vi "周期拟合倒时反应性.vi"() -> ()   [LabVIEW 2020]
uses:
  <vilib>/Utility/miscctls.llb/LVAnnotationListTypeDef.ctl
  <vilib>/Analysis/NI_AALPro.lvlib
panel:
  out "反应性相对偏差":dbl[](array[numeric]) caption="相对偏差 (%)"
  out "最小二乘周期":dbl[](array[numeric]) caption="最小二乘法拟合 (s)"
  out "广义指数周期":dbl[](array[numeric]) caption="广义指数拟合 (s)"
  out "实测平均反应性":dbl[](array[numeric]) caption="实测平均值 (pcm)"
  out "周期法反应性":dbl[](array[numeric]) caption="周期法 (pcm)"
  out "采样间隔":dbl
  out "开始时间":timestamp
  in  "打开文件":bool
  out "历史波形图":cluster{dbl, dbl, dbl[][]}(graph)
  out "左选标时刻":timestamp caption="左选标时刻：" format="%<%.2X %x>T"
  out "数据点数":i32 caption="选中的数据点数："
  out "反应性记录表":string[][](table) caption="计算结果记录表"
  in  "保存表格":bool
  in  "添加记录":bool
  out "提示信息":string="打开文件后，拖动波形图中的游标选取临界段、动态段和终端段数据进行计算。"
  out "文件信息":string
  # "周期计算结果"
  # "反应性计算结果"
  # "坐标轴与图例"
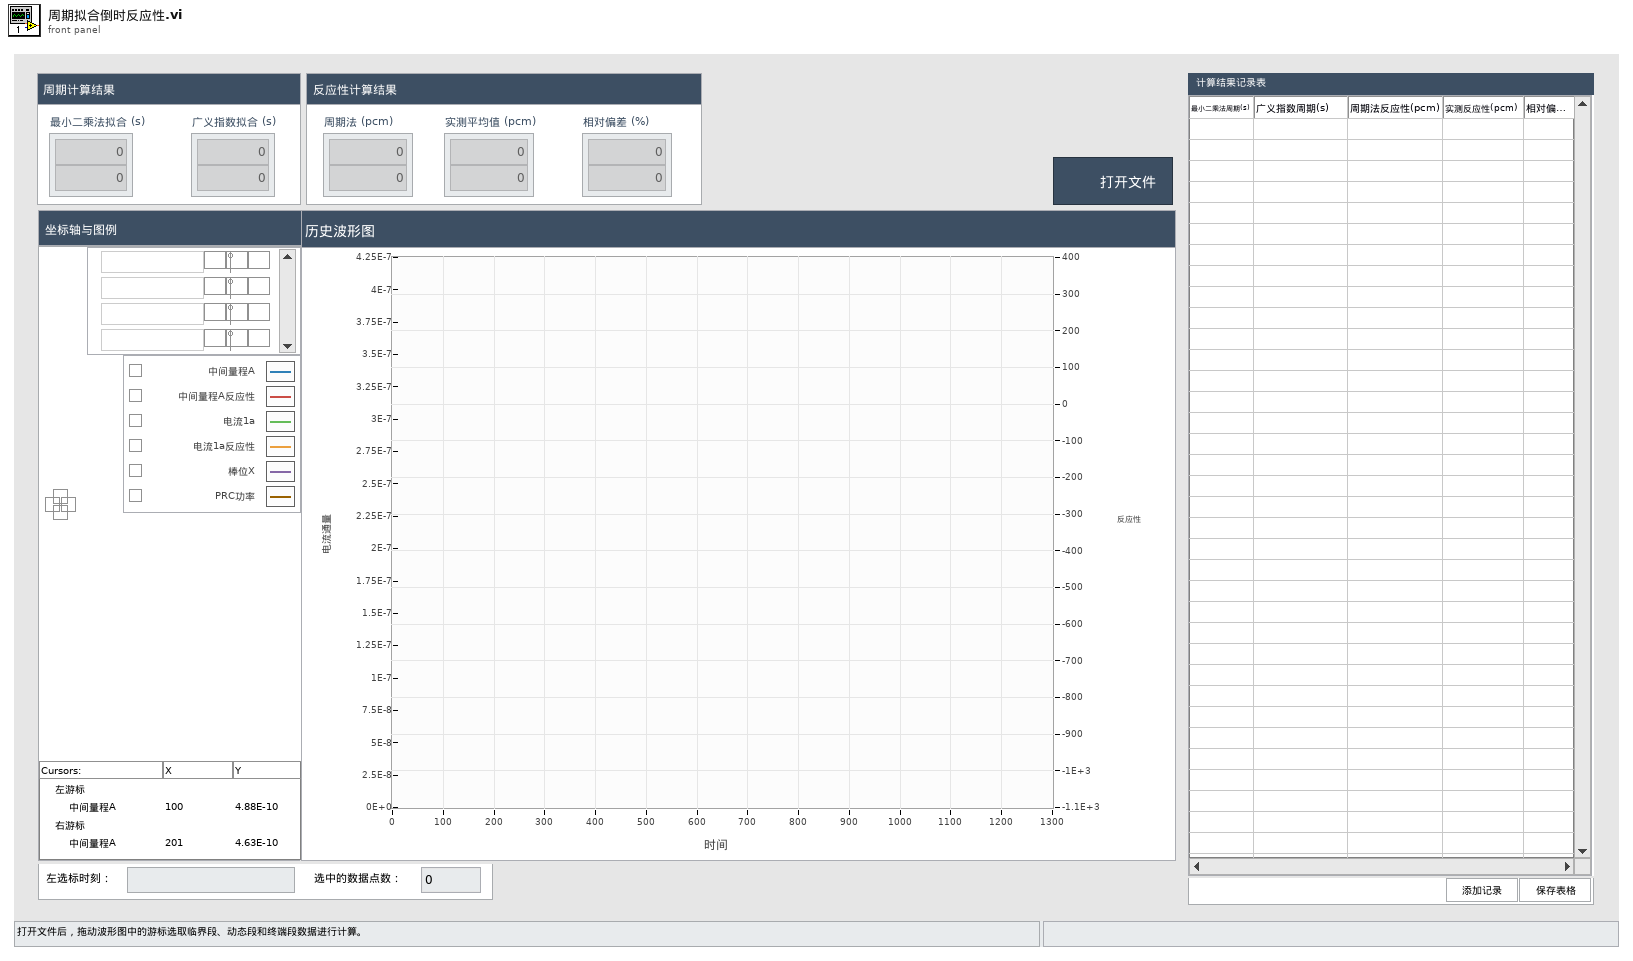
[diagram p1: front panel]
types:
  T1 = typedef "LVAnnotationListTypeDef.ctl" = cluster{"Name":string, "Color":u32, "Style":u8, "Point Style":u8, "Name Visible":bool, "Allow Drag":bool, "Annotation Mode":u32, "Plot":i32, "Index":i32, "Position":cluster{"X":dbl, "Y":dbl}, "X Scale":u32, "Y Scale":u32, "Show Arrow":bool, "Lock Name":bool, "Plot Area":i32, "Label Offset":cluster{"X":dbl, "Y":dbl}}[]
  T2 = cluster{"Name":string, "Color":u32, "Style":u8, "Point Style":u8, "Name Visible":bool, "Allow Drag":bool, "Annotation Mode":u32, "Plot":i32, "Index":i32, "Position":cluster{"X":dbl, "Y":dbl}, "X Scale":u32, "Y Scale":u32, "Show Arrow":bool, "Lock Name":bool, "Plot Area":i32, "Label Offset":cluster{"X":dbl, "Y":dbl}}
  T3 = cluster{"amp min":dbl, "amp max":dbl, "damping min":dbl, "damping max":dbl, "offset min":dbl, "offset max":dbl}
  T4 = enum16{"open", "replace", "create", "open or create", "replace or create", "replace or create with confirmation"}
  T5 = typedef "LVCursorListTypeDef.ctl" = cluster{"Name":string, "Color":u32, "Style":u8, "Point Style":u8, "Name Visible":bool, "Allow Drag":bool, "Cursor Mode":u32, "Plot":i32, "Index":i32, "Position":cluster{"X":dbl, "Y":dbl}, "X Scale":u32, "Y Scale":u32, "Watch Plots":i32[], "Watch All Plots":bool, "Plot Area":i32, "Label Offset":cluster{"X":dbl, "Y":dbl}}[]
  T6 = cluster{"Name":string, "Color":u32, "Style":u8, "Point Style":u8, "Name Visible":bool, "Allow Drag":bool, "Cursor Mode":u32, "Plot":i32, "Index":i32, "Position":cluster{"X":dbl, "Y":dbl}, "X Scale":u32, "Y Scale":u32, "Watch Plots":i32[], "Watch All Plots":bool, "Plot Area":i32, "Label Offset":cluster{"X":dbl, "Y":dbl}}
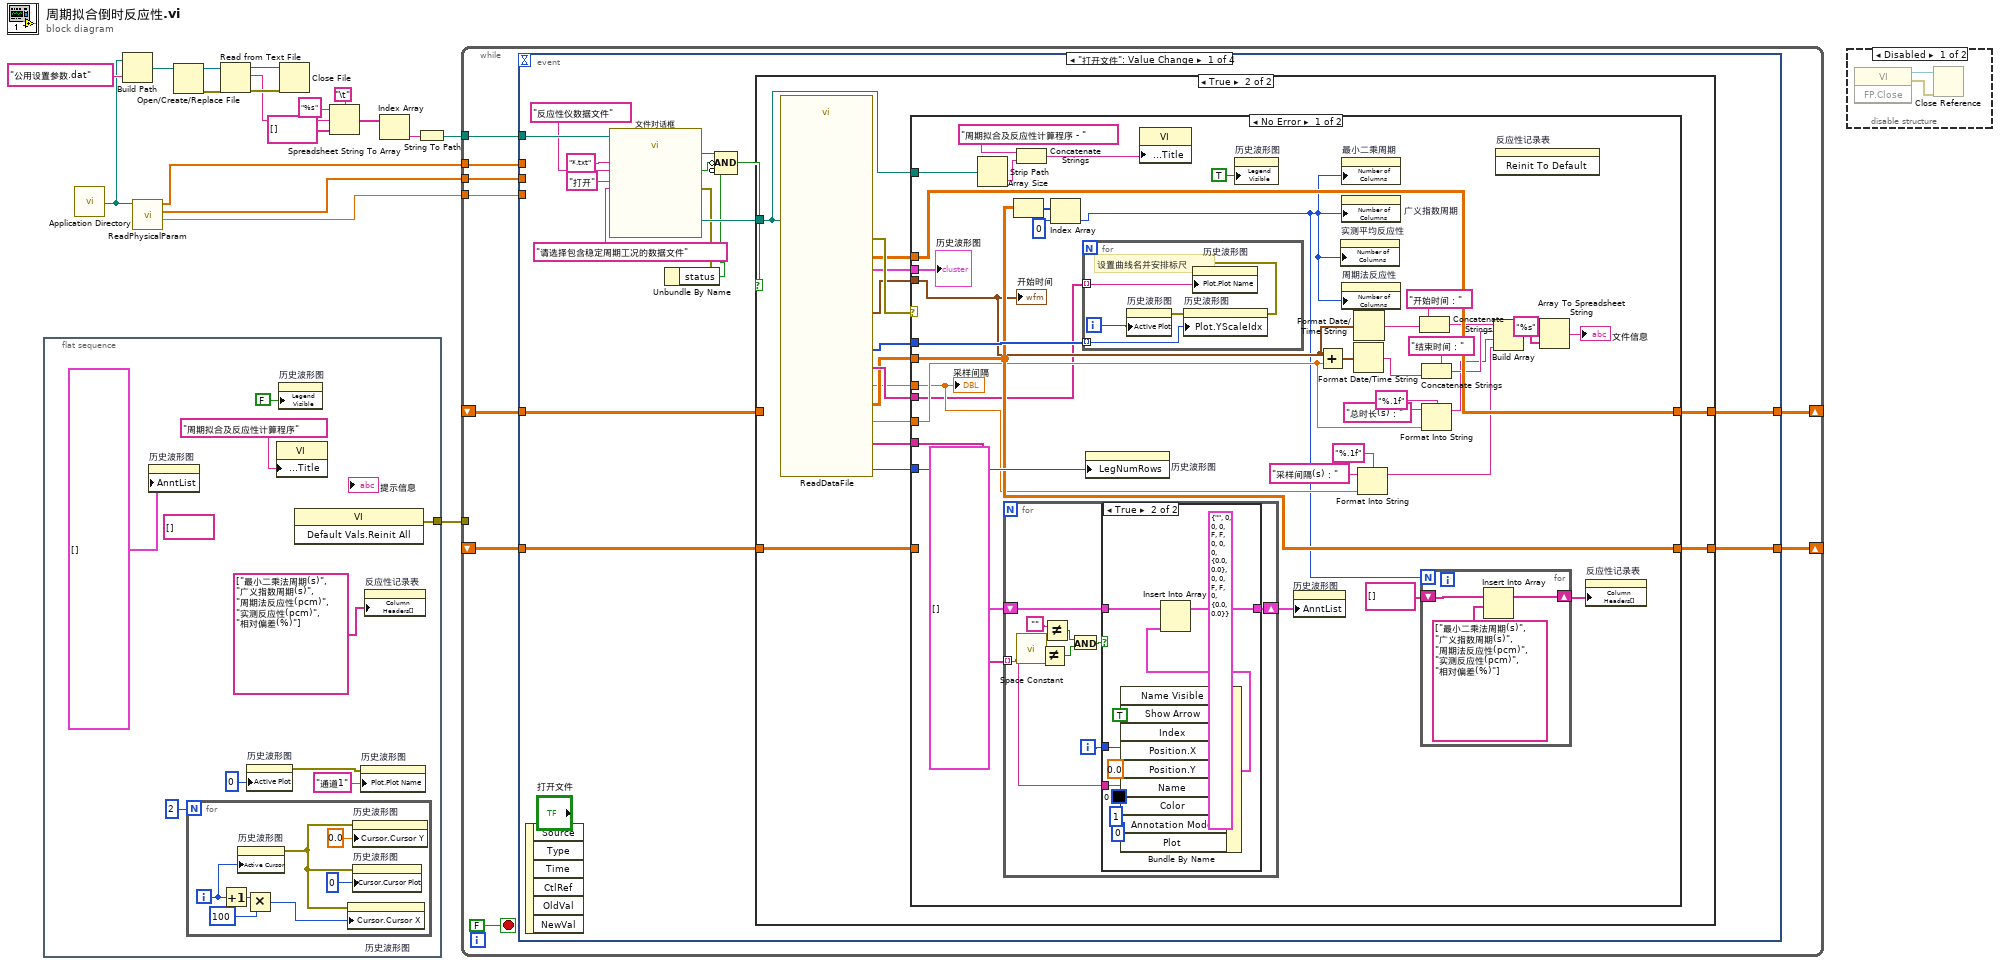
[diagram p0: block diagram]
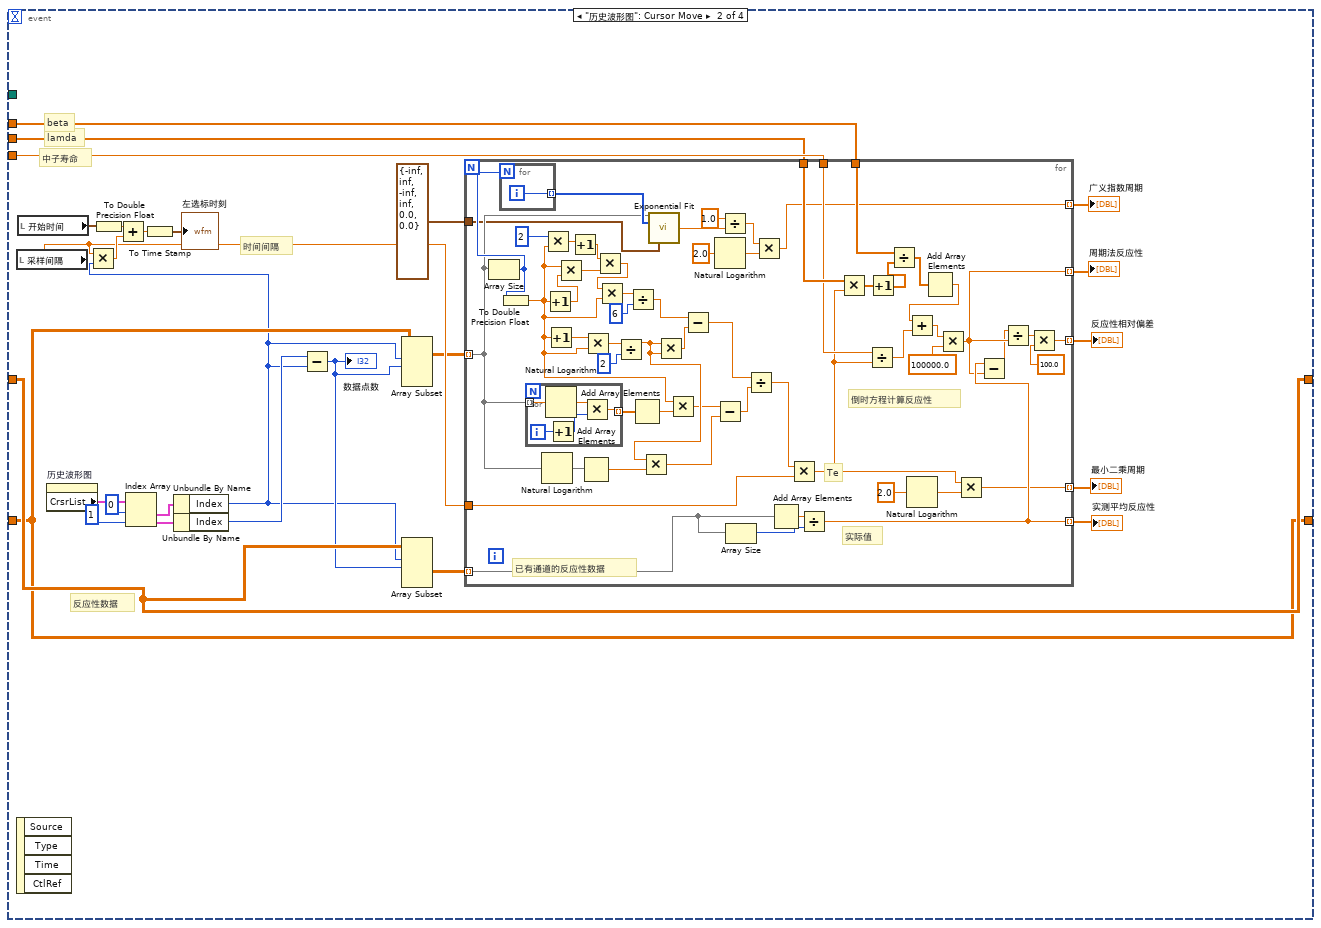
[diagram p5: hidden frame]
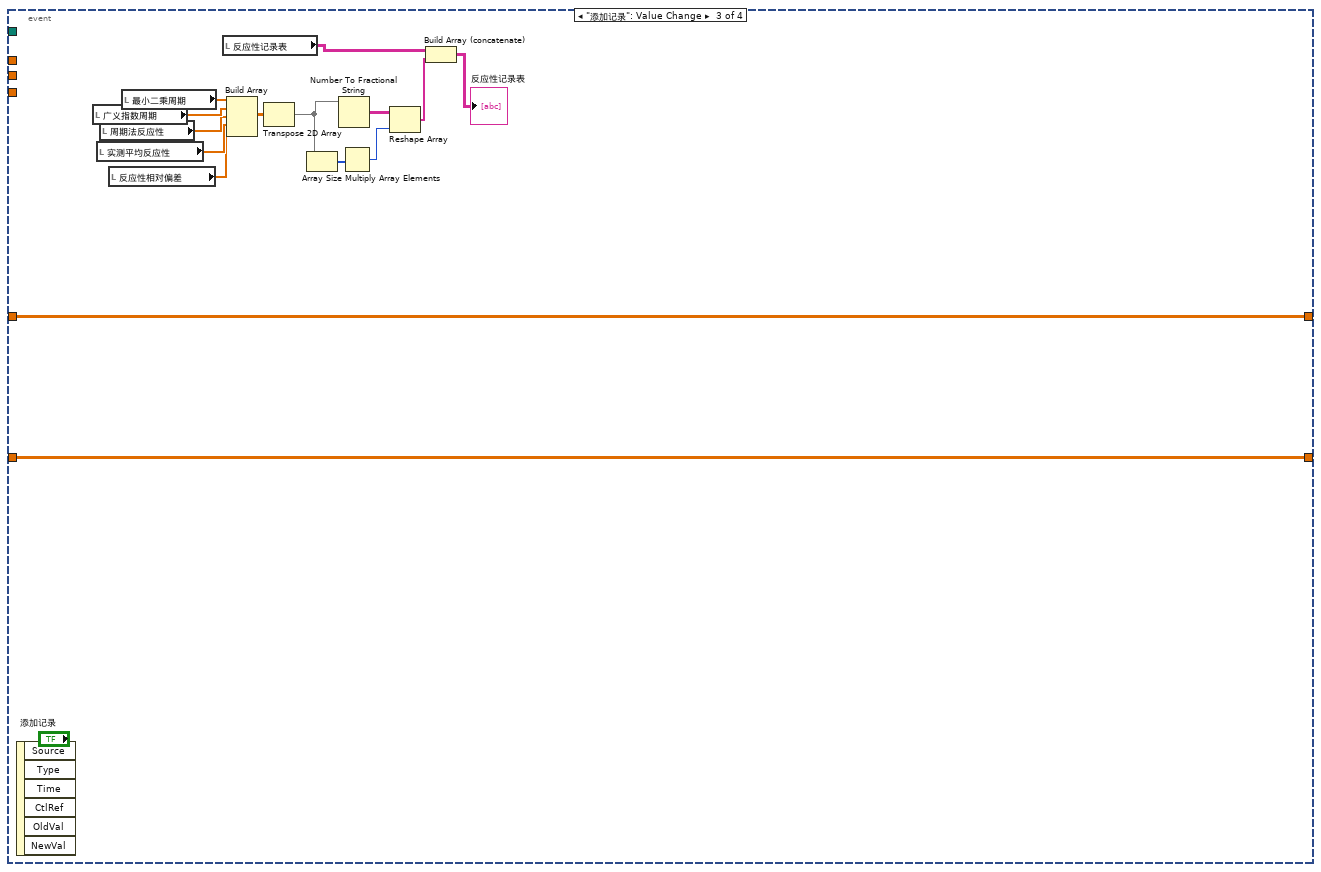
[diagram p6: hidden frame]
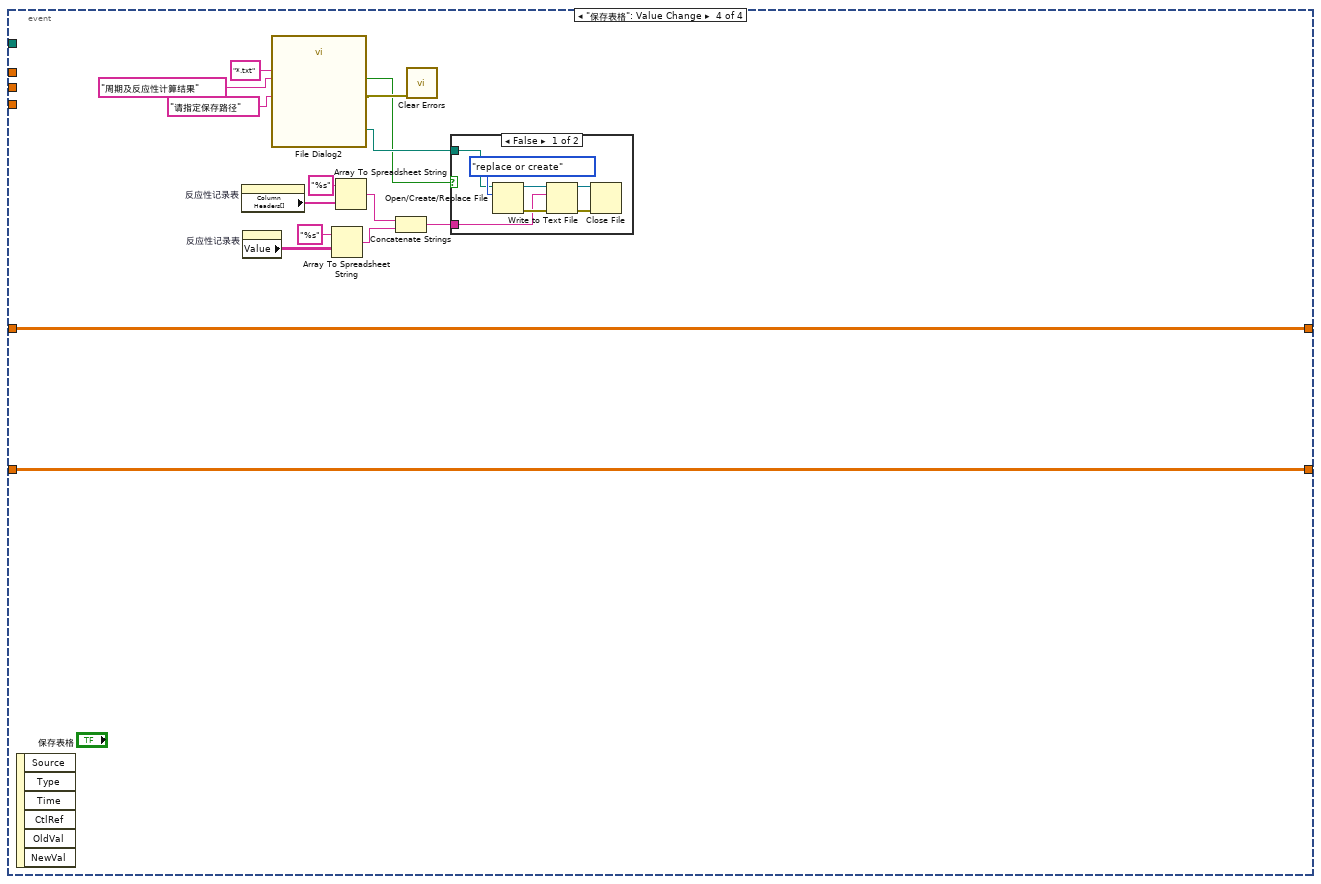
[diagram p7: hidden frame]
diagram:
  n1 = flat-sequence {
    tunnel: [w23] -> w2
    frame #0 {
      (unwired) string[] [] ("Strings []")
      n2 = property on="历史波形图" class="WFGraph (strict)"("AnntList"=T1 [] ("Annotation List")) -> ()  [unwired: 2 in, 2 out]
      n3 = for {
        N: 2 -> [_]
        i -> [w32]
        n4 = Increment(x=w32) -> (x+1=w31:i32)
        n5 = property on="历史波形图" class="WFGraph (strict)"("Active Cursor"=w32) -> (error out=w28:errorcluster)  [unwired: 2 in, 1 out]
        n6 = Multiply(x=w31, y=100) -> (x*y=w29:i32)
        n7 = property on="历史波形图" class="WFGraph (strict)"(error in=w28, "Cursor.Cursor X"=w29) -> ()  [unwired: 1 in, 2 out]
        n8 = property on="历史波形图" class="WFGraph (strict)"(error in=w28, "Cursor.Cursor Y"=0.0 ("Cursor.Cursor Position:Cursor Y")) -> ()  [unwired: 1 in, 2 out]
        n9 = property on="历史波形图" class="WFGraph (strict)"(error in=w28, "Cursor.Cursor Plot"=0 ("Cursor.Cursor Index")) -> ()  [unwired: 1 in, 2 out]
      }
      n10 = property on="历史波形图" class="WFGraph (strict)"("Active Plot"=u32 0) -> (error out=w25:errorcluster)  [unwired: 2 in, 1 out]
      n11 = property class="VI"("Front Panel.Title"="周期拟合及反应性计算程序" ("Front Panel Window:Title")) -> ()  [unwired: 2 in, 2 out]
      n12 = property on="历史波形图" class="WFGraph (strict)"("Legend Visible"=FALSE ("Legend:Visible")) -> ()  [unwired: 2 in, 2 out]
      n13 = invoke class="VI" method="Default Vals.Reinit All"() -> (error out=w23:errorcluster)  [unwired: 3 in, 2 out]
      n14 = property on="历史波形图" class="WFGraph (strict)"(error in=w25, "Plot.Plot Name"="通道1") -> ()  [unwired: 1 in, 2 out]
      n15 = property on="反应性记录表" class="Tbl (strict)"("Column Headers[]"=string[] ["最小二乘法周期(s)", "广义指数周期(s)", "周期法反应性(pcm)", "实测反应性(pcm)", "相对偏差(%)"] ("行首字符串[]")) -> ()  [unwired: 2 in, 2 out]
    }
  }
  n16 = call <vilib>:"Application Directory.vi"() -> ("Application Directory"=w1:path)
  n17 = Build Path(base path=w1, name or relative path="公用设置参数.dat") -> (appended path=w16:path)
  n18 = call "ReadPhysicalParam.vi"("堆物理参数文件路径"=w1) -> ("中子寿命(s)"=w4:sgl, "lamda"=w3:sgl[], "beta"=w5:sgl[])  [unwired: 7 in, 1 out]
  n19 = Open/Create/Replace File(file path (use dialog)=w16) -> (refnum out=w13:refnum<file>, error out=w12:errorcluster)  [unwired: 5 in, 1 out]
  n20 = Read from Text File(file (use dialog)=w13, error in=w12) -> (refnum out=w14:refnum<file>, text=w8:string, error out=w15:errorcluster)  [unwired: 1 in, 2 out]
  n21 = Close File(refnum=w14, error in=w15) -> ()  [unwired: 2 out]
  n22 = Spreadsheet String To Array(delimiter (Tab)="\t", format string="%s", spreadsheet string=w8, array type (2D Dbl)=string[] [] ("添加的数组")) -> (array=w7:string[])
  n23 = Index Array(array=w7) -> (element=w18:string)  [unwired: 1 in]
  n24 = String To Path(string=w18) -> (path=w6:path)
  n25 = while {
    tunnel: w6 -> [w43]
    shift-right: [w41] -> _
    shift-left: _ -> [w40]
    shift-right: [w39] -> _
    shift-left: _ -> [w38]
    tunnel: w5 -> [w37]
    tunnel: w4 -> [w36]
    tunnel: w3 -> [w35]
    tunnel: w2 -> [_]
    stop <- FALSE stop-if-true
    n26 = event shown="[0] \"打开文件\": Value Change" {
      selector: _ -> [_ _ _ _]
      dyn-events: _ -> [_ _ _ _]
      timeout: _ -> [_ _ _ _]
      tunnel: w43 -> [w57 _ _ _]
      tunnel: [w52 w147 w249 w264] -> w41
      tunnel: w40 -> [w51 w147 w249 w264]
      tunnel: [w50 w161 w250 w265] -> w39
      tunnel: w38 -> [w49 w161 w250 w265]
      tunnel: w37 -> [_ w152 _ _]
      tunnel: w36 -> [_ w153 _ _]
      tunnel: w35 -> [_ w151 _ _]
      event "打开文件": Value Change {
        n27 = event-data() -> ()  [unwired: 1 in, 6 out]
        n28 = call "文件对话框"("start path"=w57, "prompt"="请选择包含稳定周期工况的数据文件", "button label"="打开", "pattern (all files)"="*.txt", "pattern label"="反应性仪数据文件") -> ("selected path"=w58:path, "exists"=w47:bool, "cancelled"=w46:bool, "error out"=w48:errorcluster)  [unwired: 7 in]
        n29 = Unbundle By Name(w48) -> ("status"=w45:bool)
        n30 = Compound Arithmetic op=AND(w47, invert w46, invert w45) -> (w44:bool)
        n31 = case shown="True" w44 {
          tunnel: w58 -> [_ w61]
          tunnel: [w60 w67] -> w52
          tunnel: w51 -> [w60 w66]
          tunnel: [w59 w63] -> w50
          tunnel: w49 -> [w59 _]
          frame False {
          }
          frame True {
            n32 = call "ReadDataFile.vi"("file path (dialog if empty)"=w61) -> ("曲线对应标尺编号"=w70:i32[], "曲线名"=w69:string[], "通量数据"=w68:dbl[][], "时间间隔"=w65:dbl, "曲线数"=w72:i32, "开始时间"=w62:timestamp, "反应性数据"=w64:dbl[][], "总时长(s)"=w73:dbl, "error out"=w75:errorcluster, "备注数组"=w71:string[], "波形簇"=w74:cluster{dbl, dbl, dbl[][]})  [unwired: 2 in, 2 out]
            n33 = case shown="No Error" w75 {
              tunnel: w74 -> [w113 _]
              tunnel: w73 -> [w95 _]
              tunnel: w72 -> [w112 _]
              tunnel: w71 -> [w109 _]
              tunnel: w70 -> [w108 _]
              tunnel: w69 -> [w82 _]
              tunnel: w68 -> [w105 _]
              tunnel: [w105 w144] -> w67
              tunnel: w66 -> [_ w144]
              tunnel: w65 -> [w93 _]
              tunnel: w64 -> [w104 w143]
              tunnel: [w104 w143] -> w63
              tunnel: w62 -> [w100 _]
              tunnel: w61 -> [w77 _]
              frame No Error {
                n34 = Strip Path(path=w77) -> (name=w78:string)  [unwired: 1 out]
                n35 = for {
                  tunnel: w109 -> [w125] mode=indexing
                  shift-right: [w127] -> w111
                  shift-left: T1 [] ("注释列表") -> [w128]
                  i -> [w129]
                  n36 = call <vilib>:"Space Constant.vi"() -> ("String"=w130:string)
                  n37 = Not Equal?(x=w130, y=w125) -> (x != y?=w123:bool)
                  n38 = Not Equal?(x="", y=w125) -> (x != y?=w124:bool)
                  n39 = And(x=w124, y=w123) -> (x .and. y?=w122:bool)
                  n40 = case shown="True" w122 {
                    tunnel: w125 -> [_ w137]
                    tunnel: w129 -> [_ w139]
                    tunnel: w128 -> [w131 w142]
                    tunnel: [w131 w141] -> w127
                    frame False {
                    }
                    frame True {
                      w140 = TRUE ("Show Arrow")
                      n41 = Bundle By Name(cluster=T2 {"Name"="", "Color"=0, "Style"=0, "Point Style"=0, "Name Visible"=FALSE, "Allow Drag"=FALSE, "Annotation Mode"=0, "Plot"=0, "Index"=0, "Position"={"X"=0.0, "Y"=0.0}, "X Scale"=0, "Y Scale"=0, "Show Arrow"=FALSE, "Lock Name"=FALSE, "Plot Area"=0, "Label Offset"={"X"=0.0, "Y"=0.0}} ("元素"), "Name Visible"=w140, "Show Arrow"=w140, "Index"=w139, "Position.X"=w139, "Position.Y"=0.0 ("Y"), "Name"=w137, "Color"=u32 0, "Annotation Mode"=u32 1, "Plot"=0) -> (w138:T2)
                      n42 = Insert Into Array(array=w142, new element=w138) -> (w141:T1)  [unwired: 1 in]
                    }
                  }
                }
                n43 = Array Size(array=w105) -> (size(s)=w107:i32[])
                n44 = Concatenate Strings("周期拟合及反应性计算程序 - " ("string"), w78) -> (w79:string)
                n45 = Index Array(array=w107, index=0 ("索引")) -> (element=w81:i32)
                n46 = for {
                  tunnel: w108 -> [w119] mode=indexing
                  tunnel: w82 -> [w117] mode=indexing
                  i -> [w118]
                  # "设置曲线名并安排标尺"
                  n47 = property on="历史波形图" class="WFGraph (strict)"("Active Plot"=w118) -> (error out=w121:errorcluster)  [unwired: 2 in, 1 out]
                  n48 = property on="历史波形图" class="WFGraph (strict)"(error in=w121, "Plot.YScaleIdx"=w119) -> (error out=w120:errorcluster)  [unwired: 1 in, 1 out]
                  n49 = property on="历史波形图" class="WFGraph (strict)"(error in=w120, "Plot.Plot Name"=w117) -> ()  [unwired: 1 in, 2 out]
                }
                n50 = property on="历史波形图" class="WFGraph (strict)"("LegNumRows"=w112) -> ()  [unwired: 2 in, 2 out]
                n51 = property class="VI"("Front Panel.Title"=w79) -> ()  [unwired: 2 in, 2 out]
                n52 = property on="历史波形图" class="WFGraph (strict)"("Legend Visible"=TRUE ("Legend:Visible")) -> ()  [unwired: 2 in, 2 out]
                n53 = property on="历史波形图" class="WFGraph (strict)"("AnntList"=w111) -> ()  [unwired: 2 in, 2 out]
                n54 = Add(x=w100, y=w95) -> (x+y=w101:timestamp)
                n55 = property on="实测平均反应性" class="Arr (strict)"("Number of Columns"=w81) -> ()  [unwired: 2 in, 2 out]
                n56 = property on="最小二乘周期" class="Arr (strict)"("Number of Columns"=w81) -> ()  [unwired: 2 in, 2 out]
                n57 = property on="广义指数周期" class="Arr (strict)"("Number of Columns"=w81) -> ()  [unwired: 2 in, 2 out]
                n58 = property on="周期法反应性" class="Arr (strict)"("Number of Columns"=w81) -> ()  [unwired: 2 in, 2 out]
                n59 = Format Date/Time String(seconds (now)=w101) -> (date/time string=w96:string)  [unwired: 2 in]
                n60 = Format Date/Time String(seconds (now)=w100) -> (date/time string=w98:string)  [unwired: 2 in]
                n61 = Format Into String(format string="%.1f", initial string="采样间隔(s)：", w93) -> (resulting string=w86:string)  [unwired: 1 in, 1 out]
                n62 = Concatenate Strings("开始时间：" ("string"), w98) -> (w91:string)
                n63 = for {
                  N: w81 -> [_]
                  shift-right: [w114] -> w102
                  shift-left: string[] [] ("行首字符串[]") -> [w115]
                  n64 = Insert Into Array(array=w115, new element=string[] ["最小二乘法周期(s)", "广义指数周期(s)", "周期法反应性(pcm)", "实测反应性(pcm)", "相对偏差(%)"] ("行首字符串[]")) -> (w114:string[])  [unwired: 1 in]
                }
                n65 = Concatenate Strings("结束时间：" ("string"), w96) -> (w88:string)
                n66 = Format Into String(format string="%.1f", initial string="总时长(s)：", w95) -> (resulting string=w87:string)  [unwired: 1 in, 1 out]
                n67 = Build Array(w91, w88, w87, w86) -> (w90:string[])
                n68 = invoke on="反应性记录表" class="Tbl (strict)" method="Reinit To Default"() -> ()  [unwired: 3 in, 3 out]
                n69 = Array To Spreadsheet String(array=w90, 3:"%s" ("format string")) -> (spreadsheet string=→"文件信息":string)  [unwired: 1 in]
                n70 = property on="反应性记录表" class="Tbl (strict)"("Column Headers[]"=w102) -> ()  [unwired: 2 in, 2 out]
                "历史波形图" <- w113
                "开始时间" <- w100
                "采样间隔" <- w93
              }
              frame Error {
              }
            }
          }
        }
      }
      event "历史波形图": Cursor Move {
        # "lamda"
        # "beta"
        # "中子寿命"
        # "反应性数据"
        # "时间间隔"
        n71 = local read "采样间隔"() -> (w150:dbl)
        n72 = event-data() -> ()  [unwired: 1 in, 4 out]
        n73 = local read "开始时间"() -> (w160:timestamp)
        n74 = property on="历史波形图" class="WFGraph (strict)"() -> ("CrsrList"=w167:T5)  [unwired: 2 in, 2 out]
        n75 = To Double Precision Float(number=w160) -> (double precision float=w166:dbl)
        n76 = Index Array(array=w167, index #1=0 ("index"), index #2=1 ("index")) -> (element #1=w169:T6, element #2=w171:T6)
        n77 = Unbundle By Name(w169) -> ("Index"=w145:i32)
        n78 = Multiply(x=w150, y=w145) -> (x*y=w163:dbl)
        n79 = Add(x=w166, y=w163) -> (x+y=w165:dbl)
        n80 = To Time Stamp(1:w165) -> (0:→"左选标时刻":timestamp)
        n81 = Unbundle By Name(w171) -> ("Index"=w162:i32)
        n82 = Subtract(x=w162, y=w145) -> (x-y=w146:i32)
        "数据点数" <- w146
        n83 = Array Subset(array=w147, index (row)=w145, length (row)=w146) -> (w148:dbl[][])  [unwired: 2 in]
        n84 = Array Subset(array=w161, index (row)=w145, length (row)=w146) -> (w149:dbl[][])  [unwired: 2 in]
        n85 = for {
          tunnel: w148 -> [w180] mode=indexing
          tunnel: w153 -> [w223]
          tunnel: w152 -> [w229]
          tunnel: w151 -> [w228]
          tunnel: w149 -> [w221] mode=indexing
          tunnel: [w227] -> w157 mode=indexing
          tunnel: [w226] -> w155 mode=indexing
          tunnel: [w225] -> w154 mode=indexing
          tunnel: [w222] -> w156 mode=indexing
          tunnel: w150 -> [w224]
          tunnel: [w173] -> w158 mode=indexing
          tunnel: T3 {"amp min"=-inf, "amp max"=inf, "damping min"=-inf, "damping max"=inf, "offset min"=0.0, "offset max"=0.0} ("parameter bounds") -> [w172]
          # "已有通道的反应性数据"
          # "倒时方程计算反应性"
          # "实际值"
          # "Te"
          n86 = Array Size(array=w180) -> (size(s)=w182:i32)
          n87 = for {
            N: w182 -> [_]
            tunnel: [w230] -> w181 mode=indexing
            i -> [w230]
          }
          n88 = To Double Precision Float(number=w182) -> (double precision float=w186:dbl)
          n89 = for {
            tunnel: w180 -> [w235] mode=indexing
            tunnel: [w231] -> w198 mode=indexing
            i -> [w234]
            n90 = Natural Logarithm(1:w235) -> (0:w233:dbl)
            n91 = Increment(x=w234) -> (x+1=w232:i32)
            n92 = Multiply(x=w233, y=w232) -> (x*y=w231:dbl)
          }
          n93 = Natural Logarithm(1:w180) -> (0:w193:dbl[])
          n94 = Multiply(x=2 ("count"), y=w186) -> (x*y=w205:dbl)
          n95 = Increment(x=w186) -> (x+1=w208:dbl)
          n96 = Increment(x=w186) -> (x+1=w202:dbl)
          n97 = Multiply(x=w186, y=w208) -> (x*y=w206:dbl)
          n98 = Increment(x=w205) -> (x+1=w204:dbl)
          n99 = Add Array Elements(numeric array=w193) -> (sum=w192:dbl)
          n100 = Multiply(x=w202, y=w186) -> (x*y=w201:dbl)
          n101 = Multiply(x=w204, y=w206) -> (x*y=w203:dbl)
          n102 = Multiply(x=w203, y=w186) -> (x*y=w189:dbl)
          n103 = Divide(x=w201, y=2 ("count")) -> (x/y=w196:dbl)
          n104 = Divide(x=w189, y=6 ("count")) -> (x/y=w187:dbl)
          n105 = Add Array Elements(numeric array=w198) -> (sum=w199:dbl)
          n106 = Multiply(x=w196, y=w192) -> (x*y=w194:dbl)
          n107 = call <vilib>:"Exponential Fit.vi"("Y"=w180, "X"=w181, "parameter bounds"=w172) -> ("damping"=w178:dbl)  [unwired: 7 in, 5 out]
          n108 = Multiply(x=w196, y=w196) -> (x*y=w197:dbl)
          n109 = Multiply(x=w186, y=w199) -> (x*y=w195:dbl)
          n110 = Subtract(x=w187, y=w197) -> (x-y=w190:dbl)
          n111 = Natural Logarithm(1:sgl 2.0) -> (0:w174:sgl)
          n112 = Subtract(x=w195, y=w194) -> (x-y=w191:dbl)
          n113 = Divide(x=1.0, y=w178) -> (x/y=w175:dbl)
          n114 = Array Size(array=w221) -> (size(s)=w209:i32)
          n115 = Divide(x=w190, y=w191) -> (x/y=w179:dbl)
          n116 = Multiply(x=w175, y=w174) -> (x*y=w173:dbl)
          n117 = Add Array Elements(numeric array=w221) -> (sum=w220:dbl)
          n118 = Multiply(x=w179, y=w224) -> (x*y=w183:dbl)
          n119 = Divide(x=w220, y=w209) -> (x/y=w226:dbl)
          n120 = Multiply(x=w228, y=w183) -> (x*y=w210:dbl[])
          n121 = Divide(x=w223, y=w183) -> (x/y=w217:dbl)
          n122 = Increment(x=w210) -> (x+1=w211:dbl[])
          n123 = Divide(x=w229, y=w211) -> (x/y=w219:dbl[])
          n124 = Natural Logarithm(1:sgl 2.0) -> (0:w185:sgl)
          n125 = Add Array Elements(numeric array=w219) -> (sum=w218:dbl)
          n126 = Add(x=w218, y=w217) -> (x+y=w216:dbl)
          n127 = Multiply(x=w216, y=sgl 100000.0) -> (x*y=w225:dbl)
          n128 = Multiply(x=w183, y=w185) -> (x*y=w222:dbl)
          n129 = Subtract(x=w226, y=w225) -> (x-y=w215:dbl)
          n130 = Divide(x=w215, y=w225) -> (x/y=w214:dbl)
          n131 = Multiply(x=w214, y=sgl 100.0) -> (x*y=w227:dbl)
        }
        "周期法反应性" <- w154
        "实测平均反应性" <- w155
        "广义指数周期" <- w158
        "最小二乘周期" <- w156
        "反应性相对偏差" <- w157
      }
      event "添加记录": Value Change {
        n132 = event-data() -> ()  [unwired: 1 in, 6 out]
        n133 = local read "广义指数周期"() -> (w247:dbl[])
        n134 = local read "实测平均反应性"() -> (w245:dbl[])
        n135 = local read "周期法反应性"() -> (w246:dbl[])
        n136 = local read "反应性相对偏差"() -> (w236:dbl[])
        n137 = local read "最小二乘周期"() -> (w248:dbl[])
        n138 = local read "反应性记录表"() -> (w243:string[][])
        n139 = Build Array(w248, w247, w246, w245, w236) -> (w237:dbl[][])
        n140 = Transpose 2D Array(2D array=w237) -> (transposed array=w238:dbl[][])
        n141 = Array Size(array=w238) -> (size(s)=w240:i32[])
        n142 = Number To Fractional String(number=w238) -> (F-format string=w244:string[][])  [unwired: 3 in]
        n143 = Multiply Array Elements(1:w240) -> (0:w239:i32)
        n144 = Reshape Array(w244, w239) -> (w242:string[])
        n145 = Build Array (concatenate)(w243, w242) -> (→"反应性记录表":string[][])
      }
      event "保存表格": Value Change {
        n146 = event-data() -> ()  [unwired: 1 in, 6 out]
        n147 = property on="反应性记录表" class="Tbl (strict)"() -> ("Column Headers[]"=w263:string[])  [unwired: 2 in, 2 out]
        n148 = property on="反应性记录表" class="Tbl (strict)"() -> ("Value"=w260:string[][])  [unwired: 2 in, 2 out]
        n149 = call "File Dialog2"("prompt"="请指定保存路径" ("提示"), "pattern (all files)"="*.txt" ("类型（所有文件）"), "pattern label"="周期及反应性计算结果" ("默认名称")) -> ("selected path"=w257:path, "cancelled"=w256:bool, "error out"=w258:errorcluster)  [unwired: 9 in, 1 out]
        n150 = Array To Spreadsheet String(array=w260, 3:"%s" ("format string")) -> (spreadsheet string=w259:string)  [unwired: 1 in]
        n151 = Array To Spreadsheet String(array=w263, 3:"%s" ("格式字符串")) -> (spreadsheet string=w262:string)  [unwired: 1 in]
        n152 = Concatenate Strings(w262, w259) -> (w261:string)
        n153 = call <vilib>:"Clear Errors.vi"("error in (no error)"=w258) -> ()  [unwired: 5 in, 2 out]
        n154 = case shown="False" w256 {
          tunnel: w261 -> [w267 _]
          tunnel: w257 -> [w266 _]
          frame False {
            n155 = Open/Create/Replace File(file path (use dialog)=w266, operation (0:open)=T4."replace or create") -> (refnum out=w270:refnum<file>, error out=w272:errorcluster)  [unwired: 4 in, 1 out]
            n156 = Write to Text File(file (use dialog)=w270, text=w267, error in=w272) -> (refnum out=w269:refnum<file>, error out=w268:errorcluster)  [unwired: 1 in, 1 out]
            n157 = Close File(refnum=w269, error in=w268) -> ()  [unwired: 2 out]
          }
          frame True {
          }
        }
      }
    }
  }
  n158 = disable-structure shown="Disabled" {
    frame Disabled {
      n159 = invoke class="VI" method="FP.Close"() -> (reference out=w274:refnum<vi>, error out=w273:errorcluster)  [unwired: 3 in, 1 out]
      n160 = Close Reference(reference=w274, error in (no error)=w273) -> ()  [unwired: 1 out]
    }
    frame Enabled {
    }
  }
